vi "Set Quantity.vi"(6 "Backend engine":T1, 8 "error in":errorcluster, 11 "Quantity":T2={"Name"="A", "Value"=[[1.0]], "Uncertainty"=[[1.0]], "Degrees of Freedom"=[[10.0]], "Correlation"=[[10.0]], "Randomized uncertainty"=[[10.0]]}) -> (0 "error out":errorcluster)   [LabVIEW 2013, in "QWTBLVLib.lvlib"]
doc: "Set Quantity. Sets only non-empty arrays but array with value is always written."
uses:
  QWTBLVLib.lvlib
  TD Quantity.ctl
  TD Backend Engine.ctl
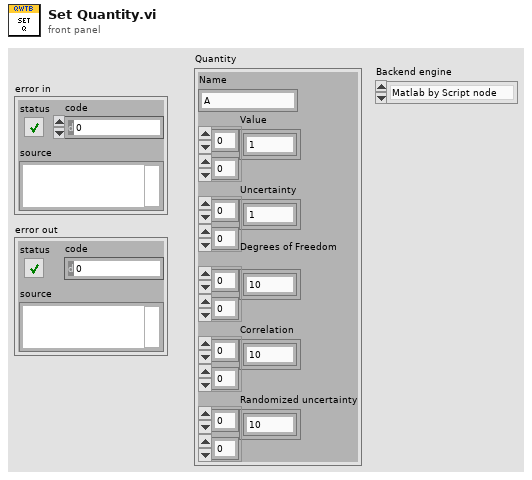
[diagram p1: front panel]
types:
  T1 = typedef "QWTBLVLib.lvlib/TD Backend Engine.ctl" = enum16{"Matlab by Script node", "GNU Octave by GOLPI"}
  T2 = typedef "QWTBLVLib.lvlib/TD Quantity.ctl" = cluster{"Name":string, "Value":dbl[][], "Uncertainty":dbl[][], "Degrees of Freedom":dbl[][], "Correlation":dbl[][], "Randomized uncertainty":dbl[][]}
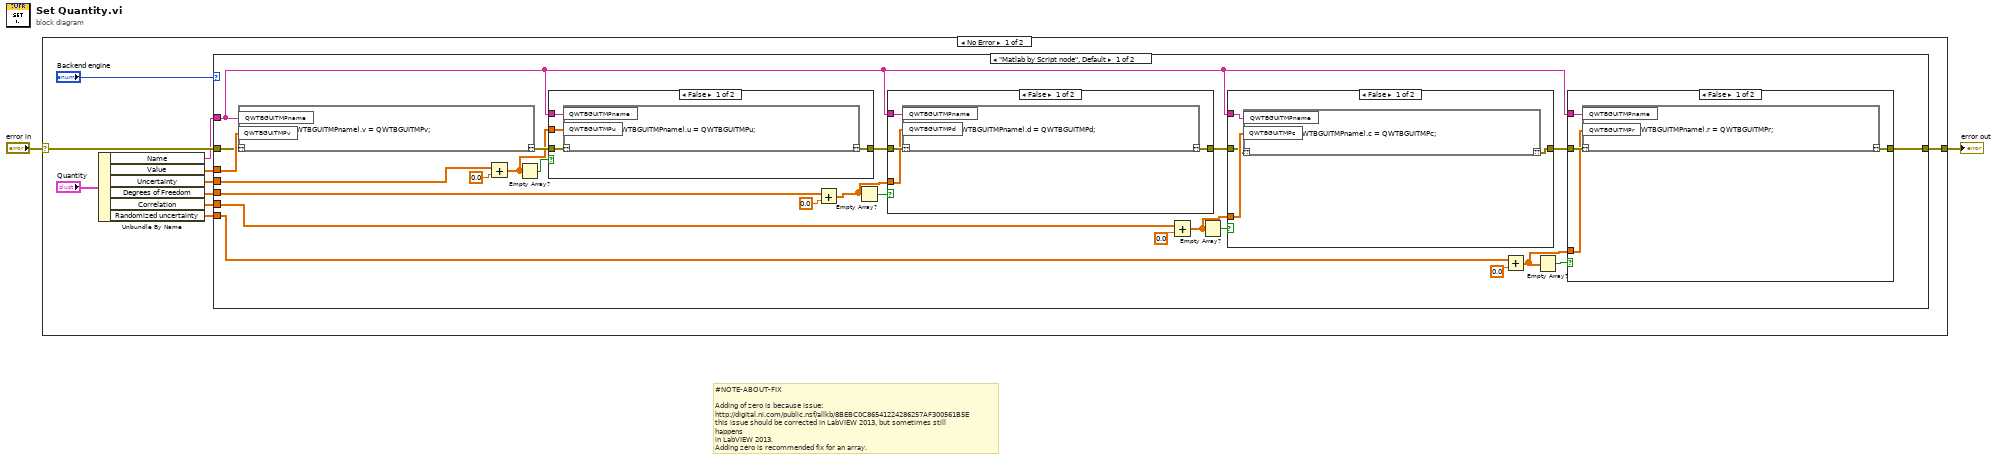
[diagram p0: block diagram]
diagram:
  # "#NOTE-ABOUT-FIX\n\nAdding of zero is because issue:\nhttp://digital.ni.com/public.nsf/allkb/8BEBC0C86541224286257AF300561B5E\nthis issue should be corrected in LabVIEW 2013, but sometimes still happens\nin LabVIEW 2013.\nAdding zero is recommended fix for an array."
  n1 = case shown="No Error" "error in" {
    selector: "error in" -> [w10 w58]
    tunnel: [w11 w58] -> w2
    frame No Error {
      n2 = Unbundle By Name("Quantity") -> ("Name"=w8:string, "Value"=w7:dbl[][], "Uncertainty"=w12:dbl[][], "Degrees of Freedom"=w6:dbl[][], "Correlation"=w5:dbl[][], "Randomized uncertainty"=w4:dbl[][])
      n3 = case shown="\"Matlab by Script node\", Default" "Backend engine" {
        tunnel: w12 -> [w17 _]
        tunnel: [w28 w57] -> w11
        tunnel: w10 -> [w25 w57]
        tunnel: w8 -> [w26 _]
        tunnel: w7 -> [w27 _]
        tunnel: w6 -> [w21 _]
        tunnel: w5 -> [w24 _]
        tunnel: w4 -> [w14 _]
        frame "Matlab by Script node", Default {
          n4 = script code="QWTBGUIdi.(QWTBGUITMPname).v = QWTBGUITMPv;"("??"=w25, "QWTBGUITMPv"=w27, "QWTBGUITMPname"=w26) -> ("??"=w35:errorcluster)
          n5 = Add(x=w17, y=0.0 ("Numeric")) -> (x+y=w16:dbl[][])
          n6 = Empty Array?(array=w16) -> (empty?=w36:bool)
          n7 = case shown="False" w36 {
            tunnel: w26 -> [w55 _]
            tunnel: w35 -> [w54 w56]
            tunnel: [w53 w56] -> w34
            tunnel: w16 -> [w52 _]
            frame False {
              n8 = script code="QWTBGUIdi.(QWTBGUITMPname).u = QWTBGUITMPu;"("??"=w54, "QWTBGUITMPu"=w52, "QWTBGUITMPname"=w55) -> ("??"=w53:errorcluster)
            }
            frame True {
            }
          }
          n9 = Add(x=w21, y=0.0 ("Numeric")) -> (x+y=w20:dbl[][])
          n10 = Empty Array?(array=w20) -> (empty?=w33:bool)
          n11 = case shown="False" w33 {
            tunnel: w26 -> [w50 _]
            tunnel: w34 -> [w49 w51]
            tunnel: [w48 w51] -> w31
            tunnel: w20 -> [w47 _]
            frame False {
              n12 = script code="QWTBGUIdi.(QWTBGUITMPname).d = QWTBGUITMPd;"("??"=w49, "QWTBGUITMPd"=w47, "QWTBGUITMPname"=w50) -> ("??"=w48:errorcluster)
            }
            frame True {
            }
          }
          n13 = Add(x=w24, y=0.0 ("Numeric")) -> (x+y=w23:dbl[][])
          n14 = Empty Array?(array=w23) -> (empty?=w32:bool)
          n15 = case shown="False" w32 {
            tunnel: w26 -> [w44 _]
            tunnel: w31 -> [w42 w46]
            tunnel: [w45 w46] -> w29
            tunnel: w23 -> [w43 _]
            frame False {
              n16 = script code="QWTBGUIdi.(QWTBGUITMPname).c = QWTBGUITMPc;"("??"=w42, "QWTBGUITMPc"=w43, "QWTBGUITMPname"=w44) -> ("??"=w45:errorcluster)
            }
            frame True {
            }
          }
          n17 = Add(x=w14, y=0.0 ("Numeric")) -> (x+y=w13:dbl[][])
          n18 = Empty Array?(array=w13) -> (empty?=w30:bool)
          n19 = case shown="False" w30 {
            tunnel: w26 -> [w40 _]
            tunnel: w29 -> [w39 w41]
            tunnel: [w38 w41] -> w28
            tunnel: w13 -> [w37 _]
            frame False {
              n20 = script code="QWTBGUIdi.(QWTBGUITMPname).r = QWTBGUITMPr;"("??"=w39, "QWTBGUITMPr"=w37, "QWTBGUITMPname"=w40) -> ("??"=w38:errorcluster)
            }
            frame True {
            }
          }
        }
        frame "GNU Octave by GOLPI" {
          # "#2do"
        }
      }
    }
    frame Error {
    }
  }
  "error out" <- w2
